vi "initializeStyle.vi"(8 "error in (no error)":errorcluster, 10 "Style":refnum<class "Style.lvclass">, 11 "xwpfRun in":refnum<class "xwpfRun.lvclass">) -> (0 "error out":errorcluster, 3 "xwpfRun out":refnum<class "xwpfRun.lvclass">)   [LabVIEW 2017, in "Word_Specific.lvlib" / "xwpfRun.lvclass"]
uses:
  xwpfRun.lvclass
  Styles/Style/Style.lvclass
  xwpfRun.lvclass/xwpfRun.ctl
  Set Style.vi
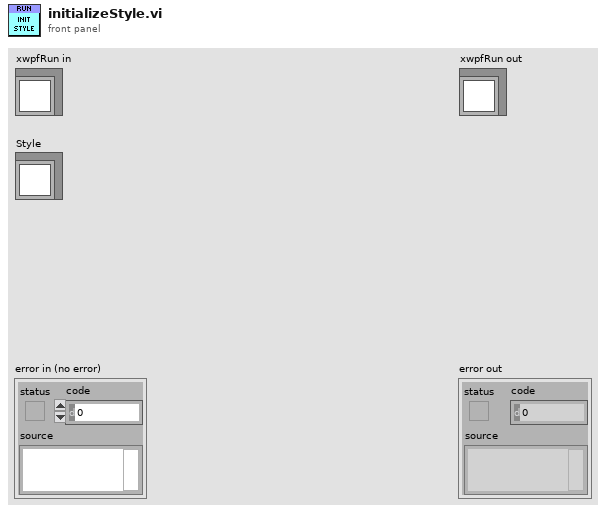
[diagram p1: front panel]
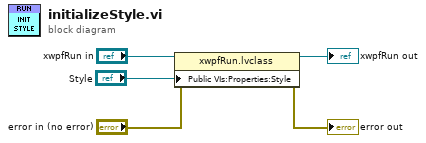
[diagram p0: block diagram]
diagram:
  n1 = property class="xwpfRun.lvclass"(reference="xwpfRun in", error in="error in (no error)", "Public VIs:Properties:Style"="Style") -> (reference out=→"xwpfRun out":refnum<class "xwpfRun.lvclass">, error out=→"error out":errorcluster)
